vi "CS-Set the inner circle parameters.vi"(0 "内圆参数in":T3={"Search  Direction"=0, "Edge Options"={"Edge Polarity"=0, "Kernel Size"=3, "Width"=3, "Minimum Edge Strength"=50.0, "Interpolation Type"=enum."Bilinear Fixed", "Data Processing Method"=enum."Average"}, "Show Search Area"=TRUE, "Show Search Lines"=TRUE, "Show Edges Found"=TRUE, "Show Result"=TRUE, "Search Area Color"=65280, "Search Lines Color"=255, "Edge Locations Color"=16776960, "Result Color"=16711680, "Overlay Group Name"=""} {"Search  Direction" items=["Outside to Inside", "Inside to Outside"]; "Edge Options"."Edge Polarity" items=["All Edges", "Rising Edges", "Falling Edges"]; "Edge Options"."Minimum Edge Strength" format="%.2f"; "Edge Options"."Width" step=2; "Edge Options"."Kernel Size" step=2}, 5 "Show Search Area":bool=TRUE, 7 "Show Search Lines":bool=TRUE, 9 "Show Edges Found":bool, 11 "Show Result":bool=TRUE) -> (4 "our":T3={"Search  Direction"=0, "Edge Options"={"Edge Polarity"=0, "Kernel Size"=3, "Width"=3, "Minimum Edge Strength"=50.0, "Interpolation Type"=enum."Bilinear Fixed", "Data Processing Method"=enum."Average"}, "Show Search Area"=TRUE, "Show Search Lines"=TRUE, "Show Edges Found"=TRUE, "Show Result"=TRUE, "Search Area Color"=65280, "Search Lines Color"=255, "Edge Locations Color"=16776960, "Result Color"=16711680, "Overlay Group Name"=""} {"Search  Direction" items=["Outside to Inside", "Inside to Outside"]; "Edge Options"."Edge Polarity" items=["All Edges", "Rising Edges", "Falling Edges"]; "Edge Options"."Minimum Edge Strength" format="%.2f"; "Edge Options"."Width" step=2; "Edge Options"."Kernel Size" step=2})   [LabVIEW 2017]
uses:
  <vilib>/vision/Measure.llb/Edge Options.ctl
  <vilib>/vision/Measure.llb/Edge Polarity.ctl
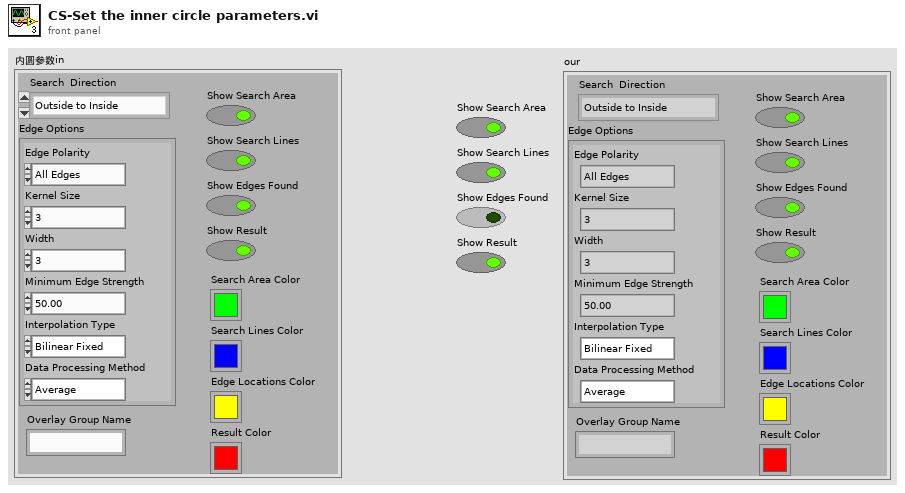
[diagram p1: front panel]
types:
  T1 = typedef "Edge Options.ctl" = cluster{"Edge Polarity":T2, "Kernel Size":u32, "Width":u32, "Minimum Edge Strength":sgl, "Interpolation Type":enum32{"Zero Order", "Bilinear", "Quadratic", "Cubic", "Bilinear Fixed"}, "Data Processing Method":enum32{"Average", "Median"}}
  T2 = typedef "Edge Polarity.ctl" = u32
  T3 = cluster{"Search  Direction":u32, "Edge Options":T1, "Show Search Area":bool, "Show Search Lines":bool, "Show Edges Found":bool, "Show Result":bool, "Search Area Color":u32, "Search Lines Color":u32, "Edge Locations Color":u32, "Result Color":u32, "Overlay Group Name":string}
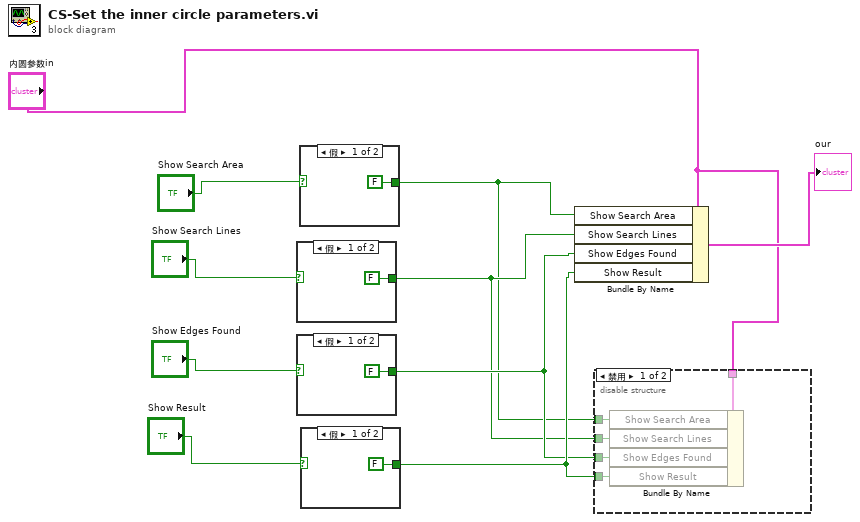
[diagram p0: block diagram]
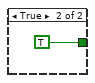
[diagram p3: hidden frame]
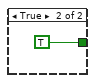
[diagram p4: hidden frame]
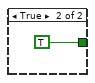
[diagram p5: hidden frame]
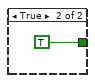
[diagram p6: hidden frame]
diagram:
  n1 = case shown="假" "Show Search Lines" {
    tunnel: [FALSE TRUE] -> w4
    frame False {
    }
    frame True {
    }
  }
  n2 = case shown="假" "Show Edges Found" {
    tunnel: [FALSE TRUE] -> w5
    frame False {
    }
    frame True {
    }
  }
  n3 = case shown="假" "Show Search Area" {
    tunnel: [FALSE TRUE] -> w3
    frame False {
    }
    frame True {
    }
  }
  n4 = case shown="假" "Show Result" {
    tunnel: [FALSE TRUE] -> w6
    frame False {
    }
    frame True {
    }
  }
  n5 = Bundle By Name(cluster="内圆参数in", "Show Search Area"=w3, "Show Search Lines"=w4, "Show Edges Found"=w5, "Show Result"=w6) -> (→"our":T3)
  n6 = disable-structure shown="禁用" {
    disable-tunnel: w6 -> [w23 _]
    disable-tunnel: w5 -> [w22 _]
    disable-tunnel: w4 -> [w21 _]
    disable-tunnel: w3 -> [w20 _]
    disable-tunnel: "内圆参数in" -> [w19 _]
    frame Disabled {
      n7 = Bundle By Name(cluster=w19, "Show Search Area"=w20, "Show Search Lines"=w21, "Show Edges Found"=w22, "Show Result"=w23) -> ()  [unwired: 1 out]
    }
    frame Enabled {
    }
  }
